vi "No Torque.vi"(7 "data":variant, 8 "qd":dbl[](array[numeric]), 9 "q":dbl[](array[numeric]), 10 "t":dbl, 11 "Robot.lvclass":refnum<class "NI_Robotics_Serial Robot Arm.lvclass">) -> (0 "error out":errorcluster, 3 "tau":dbl[](array[numeric]))   [LabVIEW 2017, in "NI_Kinematics.lvlib"]
uses:
  <vilib>/robotics/Kinematics/NI_Kinematics.lvlib
  <vilib>/robotics/Kinematics/Robot/NI_Robotics_Serial Robot Arm.lvclass
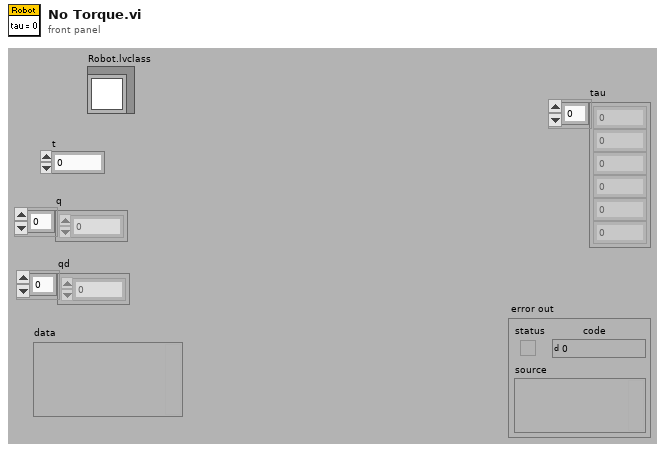
[diagram p1: front panel]
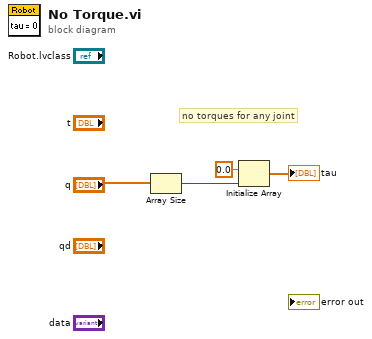
[diagram p0: block diagram]
diagram:
  # "no torques for any joint"
  n1 = Array Size(array="q") -> (size(s)=w3:i32)
  n2 = Initialize Array(0.0 ("element"), w3) -> (→"tau":dbl[])
